vi "LM model Function and gradient (Logistic Square-Gated IRF).vi"(3 "output control":T1, 4 "data":variant, 5 "X":dbl[](array[numeric]), 6 "a":dbl[](array[numeric])) -> (0 "error out":errorcluster, 1 "f'(X,a)":dbl[][](array[numeric]), 2 "f(X,a)":dbl[](array[numeric]))   [LabVIEW 2021, in "Fits.lvlib"]
doc: "This template is the starting point for creating a model function to be passed to the Nonlinear Curve Fit.vi."
uses:
  <vilib>/gmath/NumericalOptimization/LM_output select.ctl
  Fits.lvlib
  <vilib>/gmath/NI_Gmath.lvlib
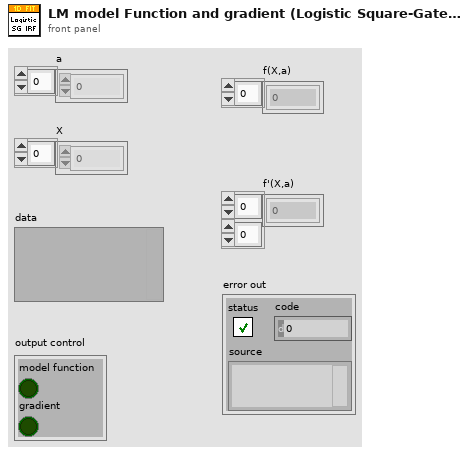
[diagram p1: front panel]
types:
  T1 = typedef "NI_Gmath.lvlib/LM_output select.ctl" = cluster{"model function":bool, "gradient":bool}
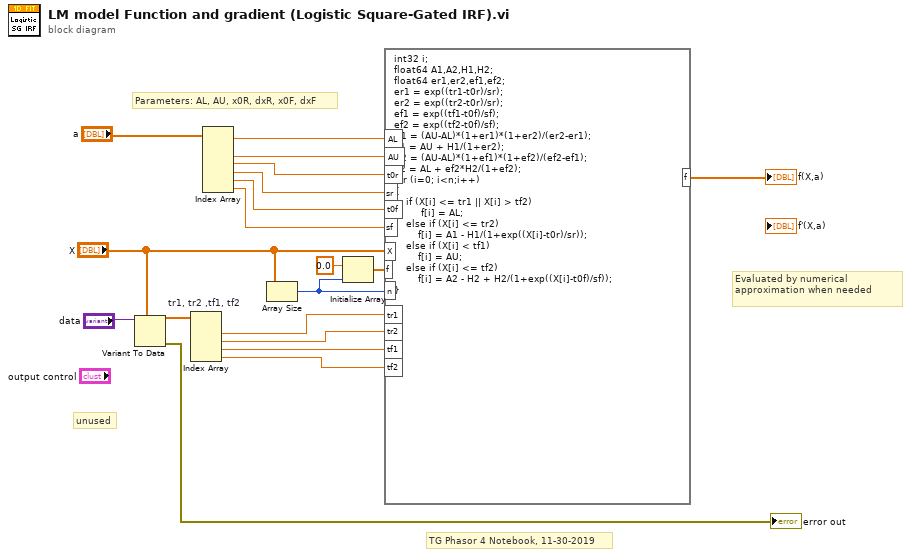
[diagram p0: block diagram]
diagram:
  # "TG Phasor 4 Notebook, 11-30-2019"
  # "Parameters: AL, AU, x0R, dxR, x0F, dxF"
  # "unused"
  # "Evaluated by numerical approximation when needed"
  n1 = Variant To Data(type="X", Variant="data") -> (data=w17:dbl[], error out=→"error out":errorcluster)  [unwired: 1 in]
  n2 = Index Array "tr1, tr2 ,tf1, tf2"(array=w17) -> (element #1=w1:dbl, element #2=w2:dbl, element #3=w3:dbl, element #4=w4:dbl)  [unwired: 4 in]
  n3 = Index Array(array="a") -> (element #1=w16:dbl, element #2=w15:dbl, element #3=w14:dbl, element #4=w13:dbl, element #5=w12:dbl, element #6=w11:dbl)  [unwired: 6 in]
  n4 = Array Size(array="X") -> (size(s)=w6:i32)
  n5 = Initialize Array(0.0 ("element"), w6) -> (w7:dbl[])
  n6 = formula code="int32 i;\nfloat64 A1,A2,H1,H2;\nfloat64 er1,er2,ef1,ef2;\ner1 = exp((tr1-t0r)/sr);\ner2 = exp((tr2-t0r)/sr);\nef1 = exp((tf1-t0f)/sf);\nef2 = exp((tf2-t0f)/sf);\nH1 = (AU-AL)*(1+er1)*(1+er2)/(er2-er1);\nA1 = AU + H1/(1+er2);\nH2 = (AU-AL)*(1+ef1)*(1+ef2)/(ef2-ef1);\nA2 = AL + ef2*H2/(1+ef2);\nfor (i=0; i<n;i++)\n{\n    if (X[i] <= tr1 || X[i] > tf2)\n         f[i] = AL;\n    else if (X[i] <= tr2)\n        f[i] = A1 - H1/(1+exp((X[i]-t0r)/sr));\n    else if (X[i] < tf1)\n        f[i] = AU;\n    else if (X[i] <= tf2)\n        f[i] = A2 - H2 + H2/(1+exp((X[i]-t0f)/sf));\n}"("AL"=w16, "AU"=w15, "X"="X", "t0r"=w14, "sr"=w13, "t0f"=w12, "sf"=w11, "tr2"=w2, "tf1"=w3, "tf2"=w4, "f"=w7, "n"=w6, "tr1"=w1) -> ("f"=→"f(X,a)":dbl[])
